vi "Check Condition.vi"(1 "Distance":dbl, 2 "Condition":dbl, 3 "Reset":bool) -> (0 "Done":bool)   [LabVIEW 2015]
uses:
  Robot Global Data.vi
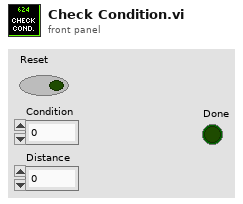
[diagram p1: front panel]
types:
  T1 = typedef "Dashboard Control Data.ctl" = cluster{"Shooter Presets":T2, "Encoder Control":T4, "Steer PID output":cluster{"output high":dbl, "output low":dbl}, " Steer PID gains":cluster{"proportional gain (Kc)":dbl, "integral time (Ti, min)":dbl, "derivative time (Td, min)":dbl}, "Drivetrain Settings":T5, "Vision Packet":T6, "Dashboard Drivetrain Command":T7, "Info/Command Cluster":T9, "Ball Vision Packet":T10, "Intake Presets":T12, "Intake Encoder Control":T14, "Climb Presets":T15, "Ultrasonic Limit":dbl, "Roll Limit":dbl, "Pitch Limit":dbl, "Goal Output Range":cluster{"output high":dbl, "output low":dbl}}
  T2 = typedef "Shooter Presets.ctl" = cluster{"Batter Shot":T3, "Deep Middle Shot":T3, "Manual Shot":T3, "Left Ticks Per Rotation":dbl, "Right Ticks Per Rotation":dbl, "Low Bar Shot":T3, "Shooter RPM Tolerance":dbl, "IIR Filter Power":dbl, "Trigger Power":dbl, "Fire from Load Delay":i32, "Angle Pot M":dbl, "Angle Pot B":dbl, "Shooter Length":dbl, "String Pot Dist":dbl, "Angle PID gains":cluster{"proportional gain (Kc)":dbl, "integral time (Ti, min)":dbl, "derivative time (Td, min)":dbl}, "Angle Motor Output":cluster{"output high":dbl, "output low":dbl}, "Shooter Angle Tolerance":dbl, "Vision Shoot x^2":dbl, "Vision Shoot x":dbl, "Dist from Axis Cam to Pivot":dbl, "High Goal Center Height":dbl, "Feed Forward Max Accel":dbl, "Feed Forward Kv":dbl, "Backwards Trigger":dbl, "Shot Finish Delay (ms)":dbl, "Angle Max Current":dbl, "Angle Current Trip Time":dbl, "Shooter Intake Angle":dbl, "Vision Shoot c":dbl, "Reset?":bool, "Servo Release Delay":dbl, "Servo Idle Angle":i32, "Servo Hold Angle":i32, "Angle Pot x^2":dbl, "Angle Pot x":dbl, "Angle Pot c":dbl}
  T3 = typedef "Shot Presets.ctl" = cluster{"Left Wheel RPM":dbl, "Right Wheel RPM":dbl, "Angle":dbl}
  T4 = typedef "Encoder Control.ctl" = cluster{"Right Tick Constant":dbl, "Left Tick Constant":dbl, "Reset?":bool, "Y Dist":cluster{"PID gains":cluster{"proportional gain (Kc)":dbl, "integral time (Ti, min)":dbl, "derivative time (Td, min)":dbl}}, "Y Stop Thresh":dbl, "Y Stop Speed":dbl}
  T5 = typedef "Drivetrain Settings.ctl" = cluster{"Gyro Tolerance":dbl, "Throttle Ramp (ms)":dbl, "Angular rate compensation":bool, "Throttle to Rate Scale":dbl, "Rate compensation gain":dbl, "Kv":dbl, "Ka":dbl, "Feed Forward P":dbl, "Feed Forward D":dbl, "Goal Vision PID gains":cluster{"proportional gain (Kc)":dbl, "integral time (Ti, min)":dbl, "derivative time (Td, min)":dbl}, "Goal Detection Window":dbl}
  T6 = typedef "Goal Vision Packet.ctl" = cluster{"Distance":dbl, "Center X":dbl, "Center Y":dbl, "Found Target?":bool}
  T7 = typedef "Dashboard Drivetrain Command.ctl" = cluster{"Drivetrain Vision":T8}
  T8 = typedef "Drivetrain Vision.ctl" = cluster{"Goal Window":dbl, "Ball Window":dbl}
  T9 = typedef "Ball Tracking Command Cluster.ctl" = cluster{"Distance to Ball":dbl, "Desired Angle":dbl, "Command":enum16{"Turn to Ball", "Turn to Angle", "Get Distance"}, "Pixels from Center":dbl}
  T10 = typedef "Ball Vision Packet.ctl" = cluster{"Ball Detected?":bool, "Distance to Ball":dbl, "Desired Angle":dbl, "Pixels from Center":dbl, "Tracking mode":T11}
  T11 = typedef "Tracking Mode.ctl" = enum16{"Turn to Ball", "Turn to Angle"}
  T12 = typedef "Intake Presets.ctl" = cluster{"Intake Speed":dbl, "Outake Speed":dbl, "Low Height":dbl, "Half Height":dbl, "Full Height":dbl, "Angle Speed":dbl, "Fast Angle":dbl, "Encoder Scale":dbl, "Load Height":dbl, "Output Range":T13, "Rotation Power Max/Min":dbl, "MaxCurrent":dbl, "Intake Trip Time":dbl, "Idle Height":dbl, "Max Height":dbl, "Reset Encoders?":bool, "PID gains":cluster{"proportional gain (Kc)":dbl, "integral time (Ti, min)":dbl, "derivative time (Td, min)":dbl}}
  T13 = typedef "Drivetrain Output Range.ctl" = cluster{"output high":dbl, "output low":dbl}
  T14 = typedef "IntakeEcoderControl.ctl" = cluster{"Arm Tick Constant":dbl, "Reset?":bool, "Y Dist":cluster{"PID gains":cluster{"proportional gain (Kc)":dbl, "integral time (Ti, min)":dbl, "derivative time (Td, min)":dbl}}, "Y Stop Thresh":dbl, "Y Stop Speed":dbl}
  T15 = typedef "Climb Presets.ctl" = cluster{"Pull Power":dbl, "Unpin Power":dbl, "Time to Hold":dbl}
  T16 = typedef "Ultrasonic Data.ctl" = cluster{"Left Ultrasonic":dbl, "Right Ultrasonic":dbl}
  T17 = typedef "IMU Data.ctl" = cluster{"Pitch":sgl, "Roll":sgl, "Yaw":sgl, "Data Valid?":bool, "Temp":sgl, "MOVING":bool, "OP Status":T18, "YAW_STABLE":bool, "Accel X":sgl, "Accel Y":sgl, "Accel Z":sgl, "Accel Magnitude":sgl, "Pitch Rate":sgl, "Roll Rate":sgl, "Yaw Rate":sgl, "NavX Opened?":bool, "Calibration Status":T19}
  T18 = typedef "navX Library v2.lvlib/Z900_navX_Flags_OpStatusTypeDef.ctl" = u8
  T19 = typedef "navX Library v2.lvlib/Z900_navX_Flags_CalibrationStatusTypeDef.ctl" = u8
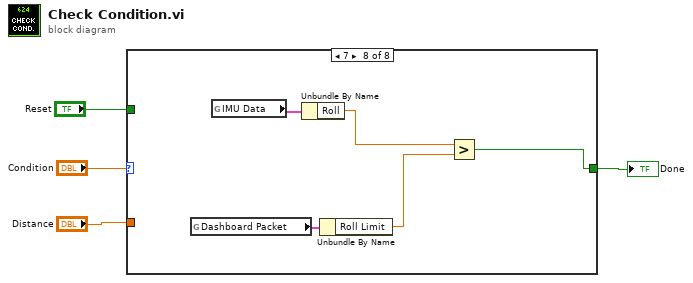
[diagram p0: block diagram]
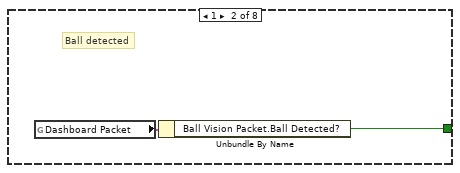
[diagram p3: hidden frame]
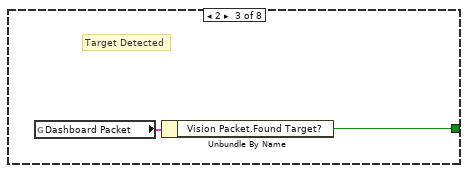
[diagram p4: hidden frame]
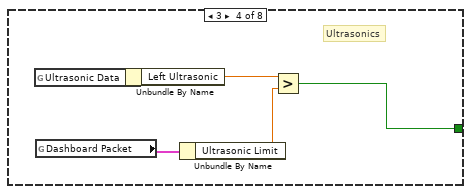
[diagram p5: hidden frame]
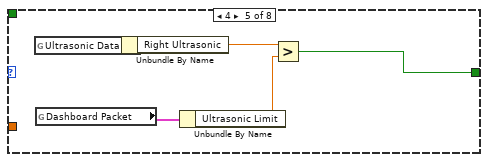
[diagram p6: hidden frame]
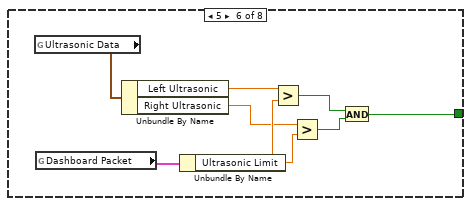
[diagram p7: hidden frame]
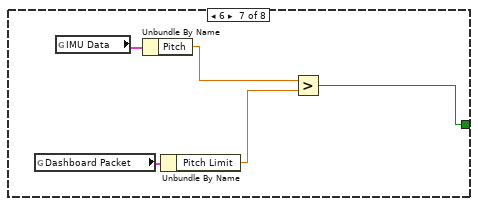
[diagram p8: hidden frame]
diagram:
  n1 = case shown="7" "Condition" {
    tunnel: "Distance" -> [_ _ _ _ _ _ _ _]
    tunnel: "Reset" -> [_ _ _ _ _ _ _ _]
    tunnel: [_ w5 w7 w12 w14 w21 w27 w32] -> w1
    frame 0, Default {
    }
    frame 1 {
      # "Ball detected"
      n2 = global read "Robot Global Data.vi" "Dashboard Packet"() -> (w6:T1)
      n3 = Unbundle By Name(w6) -> ("Ball Vision Packet.Ball Detected?"=w5:bool)
    }
    frame 2 {
      # "Target Detected"
      n4 = global read "Robot Global Data.vi" "Dashboard Packet"() -> (w8:T1)
      n5 = Unbundle By Name(w8) -> ("Vision Packet.Found Target?"=w7:bool)
    }
    frame 3 {
      # "Ultrasonics"
      n6 = global read "Robot Global Data.vi" "Ultrasonic Data"() -> (w13:T16)
      n7 = global read "Robot Global Data.vi" "Dashboard Packet"() -> (w10:T1)
      n8 = Unbundle By Name(w13) -> ("Left Ultrasonic"=w11:dbl)
      n9 = Unbundle By Name(w10) -> ("Ultrasonic Limit"=w9:dbl)
      n10 = Greater?(x=w11, y=w9) -> (0:w12:bool)
    }
    frame 4 {
      n11 = global read "Robot Global Data.vi" "Ultrasonic Data"() -> (w18:T16)
      n12 = global read "Robot Global Data.vi" "Dashboard Packet"() -> (w16:T1)
      n13 = Unbundle By Name(w18) -> ("Right Ultrasonic"=w17:dbl)
      n14 = Unbundle By Name(w16) -> ("Ultrasonic Limit"=w15:dbl)
      n15 = Greater?(x=w17, y=w15) -> (0:w14:bool)
    }
    frame 5 {
      n16 = global read "Robot Global Data.vi" "Ultrasonic Data"() -> (w26:T16)
      n17 = global read "Robot Global Data.vi" "Dashboard Packet"() -> (w24:T1)
      n18 = Unbundle By Name(w26) -> ("Left Ultrasonic"=w25:dbl, "Right Ultrasonic"=w22:dbl)
      n19 = Unbundle By Name(w24) -> ("Ultrasonic Limit"=w23:dbl)
      n20 = Greater?(x=w25, y=w23) -> (0:w20:bool)
      n21 = Greater?(x=w22, y=w23) -> (0:w19:bool)
      n22 = And(x=w20, y=w19) -> (x .and. y?=w21:bool)
    }
    frame 6 {
      n23 = global read "Robot Global Data.vi" "Dashboard Packet"() -> (w31:T1)
      n24 = global read "Robot Global Data.vi" "IMU Data"() -> (w30:T17)
      n25 = Unbundle By Name(w30) -> ("Pitch"=w29:sgl)
      n26 = Unbundle By Name(w31) -> ("Pitch Limit"=w28:dbl)
      n27 = Greater?(x=w29, y=w28) -> (0:w27:bool)
    }
    frame 7 {
      n28 = global read "Robot Global Data.vi" "Dashboard Packet"() -> (w36:T1)
      n29 = global read "Robot Global Data.vi" "IMU Data"() -> (w35:T17)
      n30 = Unbundle By Name(w35) -> ("Roll"=w34:sgl)
      n31 = Unbundle By Name(w36) -> ("Roll Limit"=w33:dbl)
      n32 = Greater?(x=w34, y=w33) -> (0:w32:bool)
    }
  }
  "Done" <- w1
